vi "sensorIdToName.vi"(8 "error in (no error)":errorcluster, 9 "Sensor ID":i32, 10 "Path":path=path "/home/ttsai/Documents/stash/ts_tcs_ofc/configData/sensorIdToName.txt", 11 "MatOper in":refnum<class "MatOper.lvclass">) -> (0 "error out":errorcluster, 2 "Sensor Name":string, 3 "MatOper out":refnum<class "MatOper.lvclass">)   [LabVIEW 2016, in "OfcFunc.lvlib" / "MatOper.lvclass"]
doc: "Map the sensor ID to name."
uses:
  MatOper.lvclass
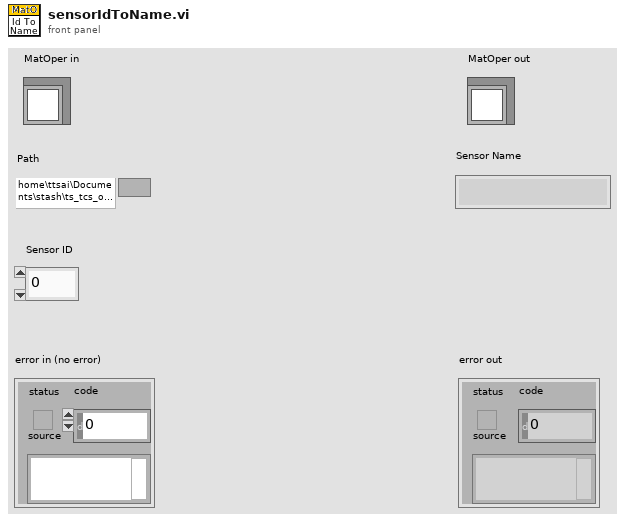
[diagram p1: front panel]
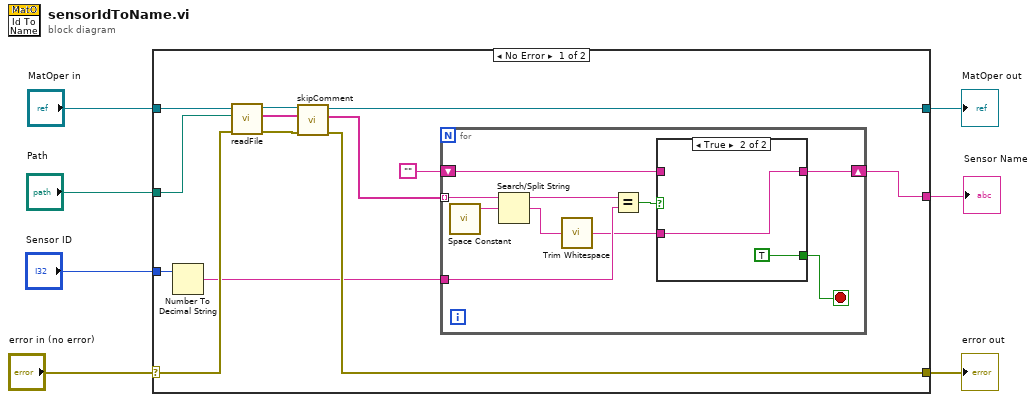
[diagram p0: block diagram]
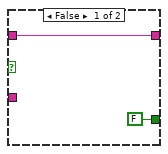
[diagram p2: hidden frame]
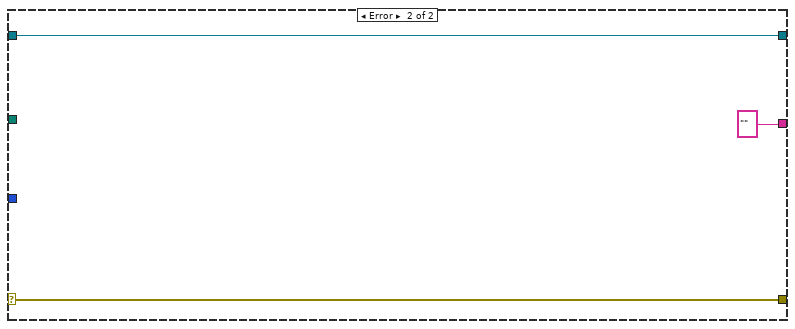
[diagram p3: hidden frame]
diagram:
  n1 = case shown="No Error" "error in (no error)" {
    selector: "error in (no error)" -> [w10 w37]
    tunnel: [w15 w37] -> w6
    tunnel: [w14 w36] -> w4
    tunnel: "MatOper in" -> [w20 w36]
    tunnel: "Path" -> [w19 _]
    tunnel: [w11 "" ("Value")] -> w2
    tunnel: "Sensor ID" -> [w8 _]
    frame No Error {
      n2 = Number To Decimal String(number=w8) -> (decimal integer string=w9:string)  [unwired: 1 in]
      n3 = call "readFile.vi"("error in (no error)"=w10, "Path"=w19, "MatOper in"=w20) -> ("error out"=w16:errorcluster, "Array"=w17:string[], "MatOper out"=w18:refnum<class "MatOper.lvclass">)  [unwired: 6 in]
      n4 = call "skipComment.vi"("error in (no error)"=w16, "Content"=w17, "MatOper in"=w18) -> ("error out"=w15:errorcluster, "Modified Content"=w13:string[], "MatOper out"=w14:refnum<class "MatOper.lvclass">)  [unwired: 6 in]
      n5 = for {
        tunnel: w13 -> [w30] mode=indexing
        tunnel: w9 -> [w26]
        shift-right: [w22] -> w11
        shift-left: "" -> [w23]
        stop <- w24 stop-if-true
        n6 = call <vilib>:"Space Constant.vi"() -> ("String"=w29:string)
        n7 = Search/Split String(string=w30, search string/char (-)=w29) -> (substring before match=w27:string, match + rest of string=w28:string)  [unwired: 1 in, 1 out]
        n8 = call <vilib>:"Trim Whitespace.vi"("string"=w28) -> ("trimmed string"=w21:string)  [unwired: 1 in]
        n9 = Equal?(x=w27, y=w26) -> (x = y?=w25:bool)
        n10 = case shown="True" w25 {
          tunnel: [FALSE TRUE] -> w24
          tunnel: w23 -> [w31 _]
          tunnel: [w31 w33] -> w22
          tunnel: w21 -> [_ w33]
          frame False {
          }
          frame True {
          }
        }
      }
    }
    frame Error {
    }
  }
  "error out" <- w6
  "MatOper out" <- w4
  "Sensor Name" <- w2
